vi "RT Driver VI.vi"(7 "Operation":T1, 11 "Device Reference in":T2 format="%.0x") -> (0 "Error Code":i32)   [LabVIEW 2016, in "FPGA Resource Manager Client Example Engine.lvlib"]
uses:
  <vilib>/NI Veristand/Custom Device API/Custom Device Item Ref.ctl
  <vilib>/NI Veristand/Custom Device API/Hardware Interface Driver VI Operation.ctl
  <vilib>/NI Veristand/Custom Device API/Custom Device Channel Type.ctl
  <vilib>/NI Veristand/Custom Device API/Data Reference.ctl
  <vilib>/NI Veristand/Custom Device API/Data Access Type.ctl
  <vilib>/NI Veristand/Custom Device API/Global Data Refs.vi
  FPGA Resource Manager Client Example Engine.lvlib
  <vilib>/NI VeriStand/Custom Device API/Custom Device API.lvlib
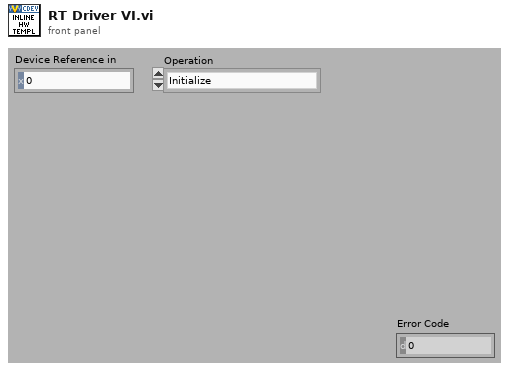
[diagram p1: front panel]
types:
  T1 = typedef "Custom Device API.lvlib/Hardware Interface Driver VI Operation.ctl" = enum16{"Initialize", "Start", "Read Data from HW", "Write Data to HW", "Close"}
  T2 = typedef "Custom Device API.lvlib/Custom Device Item Ref.ctl" = u64
  T3 = typedef "Custom Device API.lvlib/Data Reference.ctl" = i32
  T4 = cluster{"Input Values":dbl[], "Input Refs":T3[], "Output Values":dbl[], "Output Refs":T3[], "Device Error":errorcluster}
  T5 = typedef "Custom Device API.lvlib/Custom Device Channel Type.ctl" = enum16{"Input", "Output"}
  T6 = typedef "Custom Device API.lvlib/Data Access Type.ctl" = enum16{"Read", "Write"}
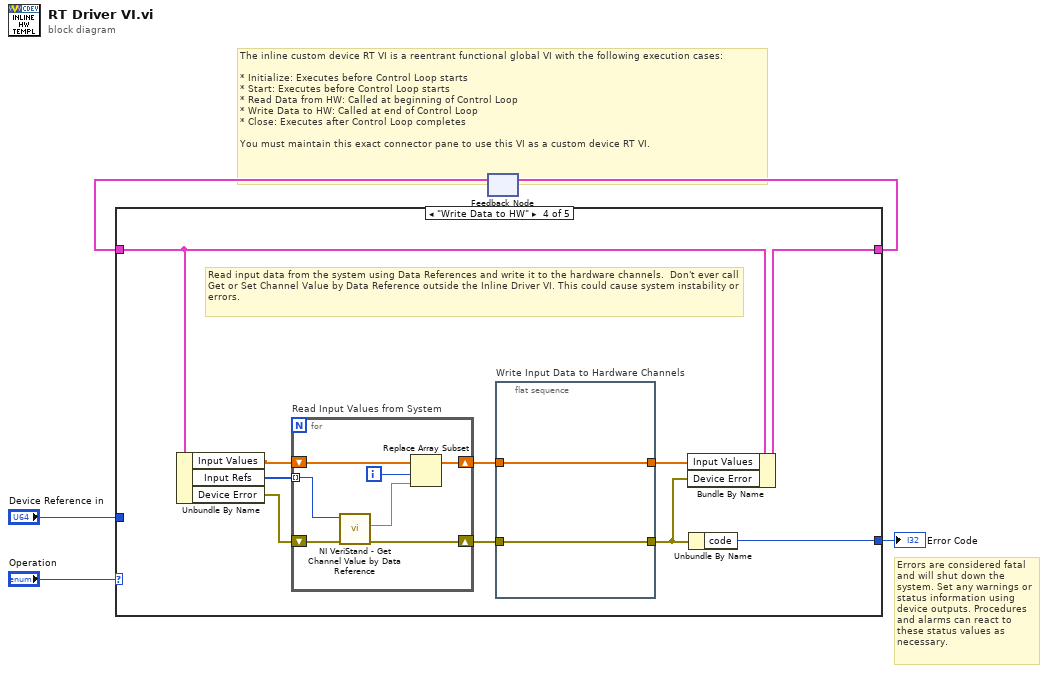
[diagram p0: block diagram]
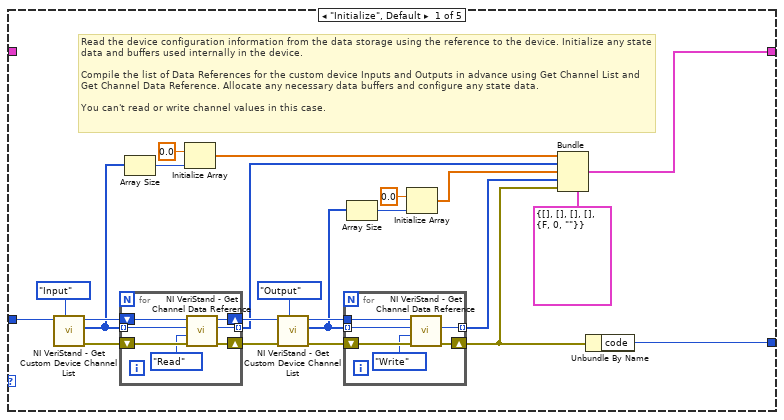
[diagram p2: hidden frame]
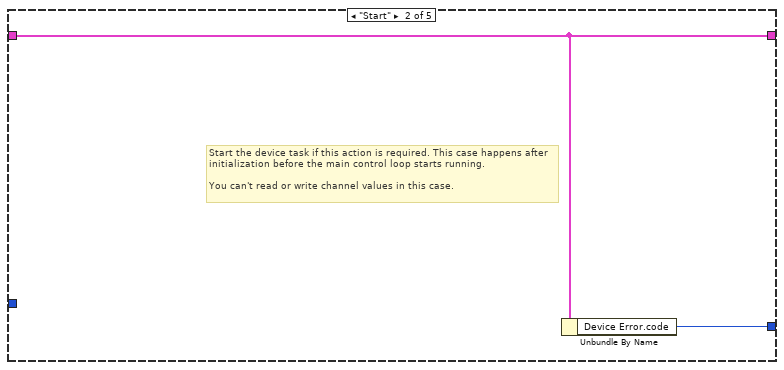
[diagram p3: hidden frame]
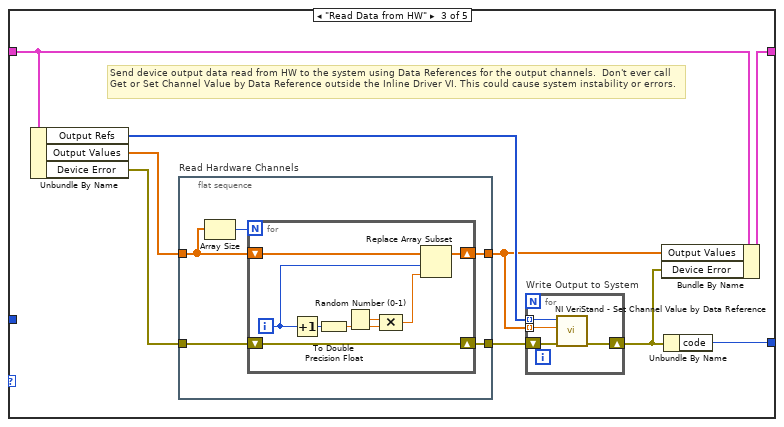
[diagram p4: hidden frame]
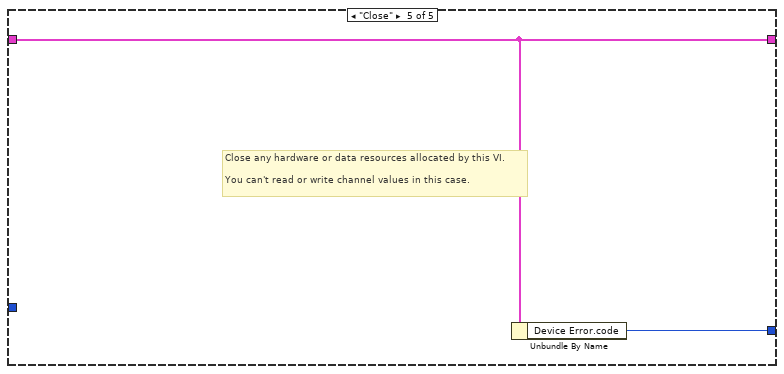
[diagram p5: hidden frame]
diagram:
  # "Errors are considered fatal and will shut down the system. Set any warnings or status information using device outputs. Procedures and alarms can react to these status values as necessary."
  # "The inline custom device RT VI is a reentrant functional global VI with the following execution cases:\n\n* Initialize: Executes before Control Loop starts\n* Start: Executes before Control Loop starts\n* Read Data from HW: Called at beginning of Control Loop\n* Write Data to HW: Called at end of Control Loop\n* Close: Executes after Control Loop completes\n\nYou must maintain this exact connector pane to use this VI as a custom device RT VI."
  n1 = feedback #1() -> (w3:T4)  [unwired: 1 out]
  n2 = case shown="\"Write Data to HW\"" "Operation" {
    tunnel: [w23 w42 w47 w78 w89] -> w4
    tunnel: w3 -> [_ w42 w48 w79 w89]
    tunnel: "Device Reference in" -> [w24 _ _ _ _]
    tunnel: [w22 w43 w51 w72 w90] -> w1
    frame "Initialize", Default {
      # "Read the device configuration information from the data storage using the reference to the device. Initialize any state data and buffers used internally in the device.\n\nCompile the list of Data References for the custom device Inputs and Outputs in advance using Get Channel List and Get Channel Data Reference. Allocate any necessary data buffers and configure any state data.\n\nYou can't read or write channel values in this case."
      n3 = call <vilib>:"NI VeriStand - Get Custom Device Channel List.vi"("Channel Type"=Custom_Device_Channel_Type."Input", "Device Ref in"=w24) -> ("error out"=w20:errorcluster, "Specified Channel Ref List"=w19:T2[], "Device Ref out"=w21:T2)  [unwired: 1 in, 6 out]
      n4 = for {
        shift-right: [w36] -> w15
        shift-left: w21 -> [w40]
        tunnel: w19 -> [w39] mode=indexing
        shift-right: [w37] -> w14
        shift-left: w20 -> [w41]
        tunnel: [w35] -> w13 mode=indexing
        n5 = call <vilib>:"NI VeriStand - Get Channel Data Reference.vi"("error in (no error)"=w41, "Access"=Data_Access_Type."Read", "Channel Ref in"=w39, "Device Ref in"=w40) -> ("error out"=w37:errorcluster, "Channel Data Reference"=w35:T3, "Device Ref out"=w36:T2)  [unwired: 5 out]
      }
      n6 = Array Size(array=w19) -> (size(s)=w27:i32)
      n7 = Initialize Array(0.0 ("element"), w27) -> (w28:dbl[])
      n8 = call <vilib>:"NI VeriStand - Get Custom Device Channel List.vi"("Channel Type"=Custom_Device_Channel_Type."Output", "error in (no error)"=w14, "Device Ref in"=w15) -> ("error out"=w18:errorcluster, "Specified Channel Ref List"=w10:T2[], "Device Ref out"=w17:T2)  [unwired: 6 out]
      n9 = for {
        tunnel: w10 -> [w32] mode=indexing
        shift-right: [w30] -> w6
        shift-left: w18 -> [w34]
        tunnel: [w29] -> w8 mode=indexing
        tunnel: w17 -> [w33]
        n10 = call <vilib>:"NI VeriStand - Get Channel Data Reference.vi"("error in (no error)"=w34, "Access"=Data_Access_Type."Write", "Channel Ref in"=w32, "Device Ref in"=w33) -> ("error out"=w30:errorcluster, "Channel Data Reference"=w29:T3)  [unwired: 6 out]
      }
      n11 = Array Size(array=w10) -> (size(s)=w11:i32)
      n12 = Initialize Array(0.0 ("element"), w11) -> (w9:dbl[])
      n13 = Bundle(cluster=T4 {"Input Values"=[], "Input Refs"=[], "Output Values"=[], "Output Refs"=[], "Device Error"={"status"=FALSE, "code"=0, "source"=""}}, "Input Values"=w28, "Input Refs"=w13, "Output Values"=w9, "Output Refs"=w8, "Device Error"=w6) -> (w23:T4)
      n14 = Unbundle By Name(w6) -> ("code"=w22:i32)
    }
    frame "Start" {
      # "Start the device task if this action is required. This case happens after initialization before the main control loop starts running.\n\nYou can't read or write channel values in this case."
      n15 = Unbundle By Name(w42) -> ("Device Error.code"=w43:i32)
    }
    frame "Read Data from HW" {
      # "Send device output data read from HW to the system using Data References for the output channels.  Don't ever call Get or Set Channel Value by Data Reference outside the Inline Driver VI. This could cause system instability or errors."
      n16 = Unbundle By Name(w48) -> ("Output Refs"=w50:T3[], "Output Values"=w49:dbl[], "Device Error"=w45:errorcluster)
      n17 = flat-sequence "Read Hardware Channels" {
        tunnel: w45 -> [w61]
        tunnel: [w60] -> w52
        tunnel: [w57] -> w46
        tunnel: w49 -> [w58]
        frame #0 {
          n18 = Array Size(array=w58) -> (size(s)=w59:i32)
          n19 = for {
            N: w59 -> [_]
            shift-right: [w66] -> w60
            shift-left: w61 -> [w66]
            shift-right: [w63] -> w57
            shift-left: w58 -> [w65]
            i -> [w62]
            n20 = Increment(x=w62) -> (x+1=w68:i32)
            n21 = To Double Precision Float(number=w68) -> (double precision float=w67:dbl)
            n22 = Random Number (0-1)() -> (number: 0 to 1=w69:dbl)
            n23 = Compound Arithmetic op=MULTIPLY(w69, w67) -> (w64:dbl)
            n24 = Replace Array Subset(array=w65, new element=w64, index=w62) -> (w63:dbl[])
          }
        }
      }
      n25 = for "Write Output to System" {
        shift-right: [w55] -> w44
        shift-left: w52 -> [w56]
        tunnel: w46 -> [w54] mode=indexing
        tunnel: w50 -> [w53] mode=indexing
        n26 = call <vilib>:"NI VeriStand - Set Channel Value by Data Reference.vi"("error in (no error)"=w56, "Value"=w54, "Data Reference in"=w53) -> ("error out"=w55:errorcluster)  [unwired: 8 out]
      }
      n27 = Bundle By Name(cluster=w48, "Output Values"=w46, "Device Error"=w44) -> (w47:T4)
      n28 = Unbundle By Name(w44) -> ("code"=w51:i32)
    }
    frame "Write Data to HW" {
      # "Read input data from the system using Data References and write it to the hardware channels.  Don't ever call Get or Set Channel Value by Data Reference outside the Inline Driver VI. This could cause system instability or errors."
      n29 = Unbundle By Name(w79) -> ("Input Values"=w76:dbl[], "Input Refs"=w77:T3[], "Device Error"=w71:errorcluster)
      n30 = for "Read Input Values from System" {
        shift-right: [w82] -> w73
        shift-left: w71 -> [w88]
        tunnel: w77 -> [w87] mode=indexing
        shift-right: [w85] -> w75
        shift-left: w76 -> [w86]
        i -> [w84]
        n31 = call <vilib>:"NI VeriStand - Get Channel Value by Data Reference.vi"("error in (no error)"=w88, "Data Reference in"=w87) -> ("error out"=w82:errorcluster, "Value"=w83:dbl)  [unwired: 8 out]
        n32 = Replace Array Subset(array=w86, new element=w83, index=w84) -> (w85:dbl[])
      }
      n33 = flat-sequence "Write Input Data to Hardware Channels" {
        tunnel: w75 -> [w81]
        tunnel: [w81] -> w74
        tunnel: [w80] -> w70
        tunnel: w73 -> [w80]
        frame #0 {
        }
      }
      n34 = Bundle By Name(cluster=w79, "Input Values"=w74, "Device Error"=w70) -> (w78:T4)
      n35 = Unbundle By Name(w70) -> ("code"=w72:i32)
    }
    frame "Close" {
      # "Close any hardware or data resources allocated by this VI.\n\nYou can't read or write channel values in this case."
      n36 = Unbundle By Name(w89) -> ("Device Error.code"=w90:i32)
    }
  }
  "Error Code" <- w1
  n37 = feedback-in #1(w4) -> ()
